vi "OSF Create Component.vi"(7 "OSF API URL":string="https://api.osf.io/v2/", 8 "error in":errorcluster, 9 "Child name":string, 10 "Parent  ID":string, 11 "client handle":T2) -> (0 "error out":errorcluster, 2 "Component ID":string caption="Project ID", 3 "client handle out":T2)   [LabVIEW 2020]
uses:
  <vilib>/httpClient/ClientHandle.ctl
  55103850-15ef-4a18-9388-7b0eadcdd449.vi
  <vilib>/JDP Science/JSONtext/Variant to JSON Text.vi
  <vilib>/httpClient/POSTBuffer.vi
  <vilib>/httpClient/LabVIEWHTTPClient.lvlib
panel:
  out "Responce body":string
  in  "OSF child":T1={"data"={"type"="nodes", "attributes"={"title"="", "description"="", "public"=FALSE, "category"="project"}}}
  out "Puject  JSON":string
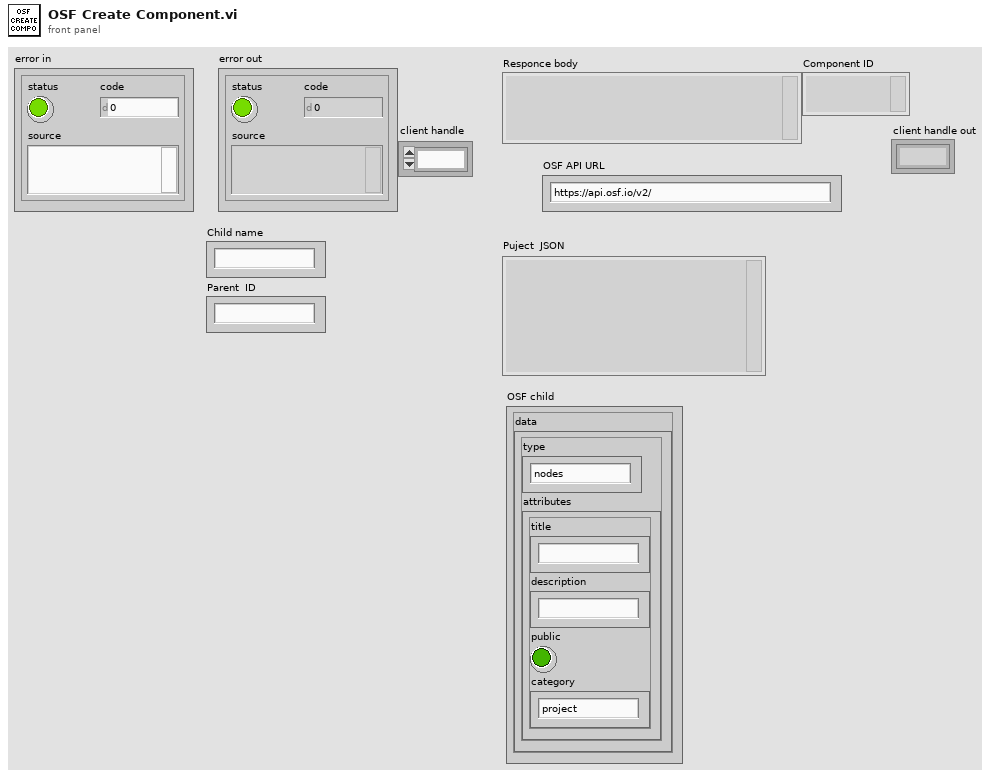
[diagram p1: front panel]
types:
  T1 = cluster{"data":cluster{"type":string, "attributes":cluster{"title":string, "description":string, "public":bool, "category":string}}}
  T2 = typedef "LabVIEWHTTPClient.lvlib/ClientHandle.ctl" = refnum<k1>
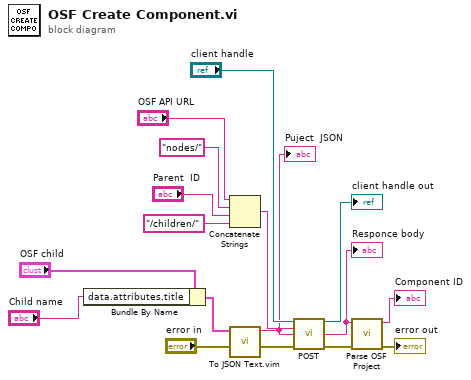
[diagram p0: block diagram]
diagram:
  n1 = Bundle By Name(cluster="OSF child", "data.attributes.title"="Child name") -> (w17:T1)
  n2 = Concatenate Strings("OSF API URL", "nodes/", "Parent  ID", "/children/" ("string")) -> (w8:string)
  n3 = call "To JSON Text.vim"("error in (no error)"="error in", "Anything"=w17) -> ("error out"=w7:errorcluster, "<JSON>"=w5:string)  [unwired: 8 in]
  "Puject  JSON" <- w5
  n4 = call-poly <vilib>:"POST.vi"("client handle"="client handle", "url"=w8, "buffer"=w5, "error in (no error)"=w7) -> ("client handle out"=→"client handle out":T2, "body"=w2:string, "error out"=w4:errorcluster)  [unwired: 8 in, 1 out]
  "Responce body" <- w2
  n5 = call "Parse OSF Project.vi"("error in"=w4, "Project JSON"=w2) -> ("error out"=→"error out":errorcluster, "Project ID"=→"Component ID":string)  [unwired: 7 in, 1 out]
